vi "Demo.vi"() -> ()   [LabVIEW 2011]
uses:
  StatD Class/Controls/Event Types.ctl
  StatD Class/StatD Interface.lvclass
panel:
  in  "Send Event":bool
  in  "Event Type (info)":T1=enum."info"
  in  "Event Text":string
  in  "Event Title":string
  in  "stop":bool
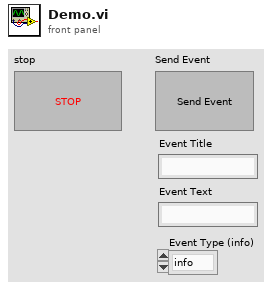
[diagram p1: front panel]
types:
  T1 = typedef "StatD Interface.lvclass/Event Types.ctl" = enum16{"error", "warning", "info", "success"}
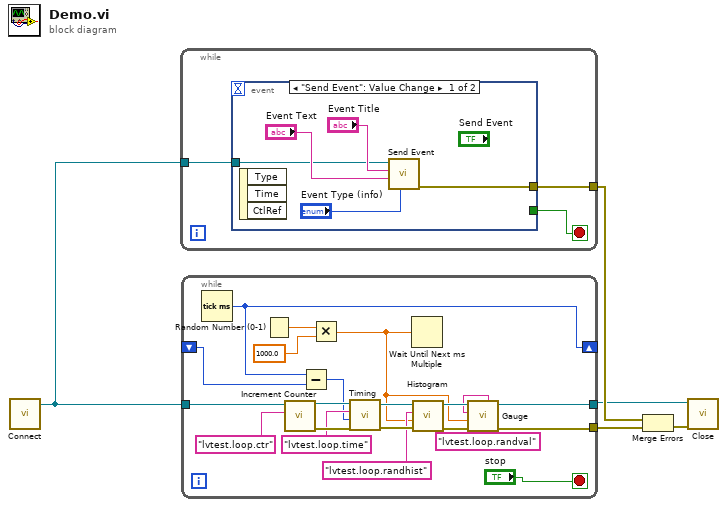
[diagram p0: block diagram]
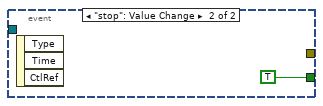
[diagram p2: hidden frame]
diagram:
  n1 = call "Connect.vi"() -> ("StatD Interface out"=w5:refnum<class "StatD Interface.lvclass">)  [unwired: 10 in, 1 out]
  n2 = while {
    tunnel: w5 -> [w7]
    tunnel: [w6] -> w4
    stop <- w8 stop-if-true
    n3 = event shown="[0] \"Send Event\": Value Change" {
      selector: _ -> [_ _]
      dyn-events: _ -> [_ _]
      timeout: _ -> [_ _]
      tunnel: [_ TRUE] -> w8
      tunnel: w7 -> [w10 _]
      tunnel: [w9 _] -> w6
      event "Send Event": Value Change {
        n4 = event-data() -> ()  [unwired: 1 in, 3 out]
        n5 = call "Send Event.vi"("Event Type (info)"="Event Type (info)", "Event Text"="Event Text", "Event Title"="Event Title", "StatD Interface in"=w10) -> ("error out"=w9:errorcluster)  [unwired: 6 in, 1 out]
      }
      event "stop": Value Change {
        n6 = event-data() -> ()  [unwired: 1 in, 3 out]
      }
    }
  }
  n7 = while {
    tunnel: w5 -> [w31]
    shift-right: [w26] -> _
    shift-left: _ -> [w25]
    tunnel: [w16] -> w1
    tunnel: [w15] -> w3
    stop <- "stop" stop-if-true
    n8 = Tick Count (ms)() -> (millisecond timer value=w26:u32)
    n9 = Random Number (0-1)() -> (number: 0 to 1=w33:dbl)
    n10 = call "Increment Counter.vi"("Metric Name"="lvtest.loop.ctr", "StatD Interface in"=w31) -> ("error out"=w29:errorcluster, "StatD Interface out"=w28:refnum<class "StatD Interface.lvclass">)  [unwired: 8 in]
    n11 = Subtract(x=w26, y=w25) -> (x-y=w24:u32)
    n12 = Multiply(x=w33, y=1000.0) -> (x*y=w17:dbl)
    n13 = call "Timing.vi"("error in (no error)"=w29, "Time (ms)"=w24, "Metric Name"="lvtest.loop.time", "StatD Interface in"=w28) -> ("error out"=w22:errorcluster, "StatD Interface out"=w23:refnum<class "StatD Interface.lvclass">)  [unwired: 6 in]
    n14 = Wait Until Next ms Multiple(millisecond multiple=w17) -> ()  [unwired: 1 out]
    n15 = call "Histogram.vi"("error in (no error)"=w22, "Metric Value"=w17, "Metric Name"="lvtest.loop.randhist", "StatD Interface in"=w23) -> ("error out"=w20:errorcluster, "StatD Interface out"=w21:refnum<class "StatD Interface.lvclass">)  [unwired: 6 in]
    n16 = call "Gauge.vi"("error in (no error)"=w20, "Metric Value"=w17, "Metric Name"="lvtest.loop.randval", "StatD Interface in"=w21) -> ("error out"=w15:errorcluster, "StatD Interface out"=w16:refnum<class "StatD Interface.lvclass">)  [unwired: 6 in]
  }
  n17 = Merge Errors(w4, w3) -> (w2:errorcluster)
  n18 = call "Close.vi"("error in (no error)"=w2, "StatD Interface in"=w1) -> ()  [unwired: 9 in, 1 out]
